vi "WPI_CameraSet Exposure Priority.vi"(8 "error in (no error)":errorcluster, 10 "Exposure Priority":T2, 11 "CameraDevRef":T1={"Camera Address"="192.168.0.90", "CameraStatus"={"status"=FALSE, "code"=0, "source"=""}}) -> (0 "error out":errorcluster, 3 "CameraDevRef Out":T1)   [LabVIEW 2017]
doc: "Specifies whether the camera you specify prioritizes the frame rate or image quality when setting the exposure.\n\nThis software is licensed. Open the labview\\readme\\WPI Robotics Library Open Source License.txt file for more information."
uses:
  <vilib>/Rock Robotics/WPI/Camera/WPI_CameraExposure Priority Values.ctl
  <vilib>/Rock Robotics/WPI/Camera/WPI_CameraDevRef.ctl
  <vilib>/Rock Robotics/WPI/Camera/WPI_CameraSettings Operations.ctl
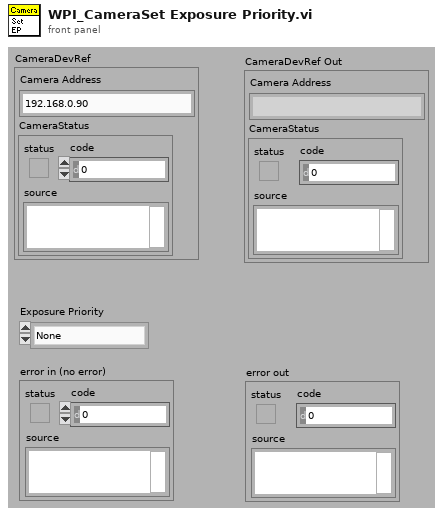
[diagram p1: front panel]
types:
  T1 = typedef "WPI_CameraDevRef.ctl" = cluster{"Camera Address":string, "CameraStatus":errorcluster}
  T2 = typedef "WPI_CameraExposure Priority Values.ctl" = enum16{"None", "Prioritize frame rate", "Prioritize image quality"}
  T3 = typedef "WPI_CameraSettings Operations.ctl" = enum16{"Udate FPS", "Update Compression", "Update Size", "Update White Balance", "Update Brightness", "Update Sharpness", "Update Exposure", "Update Exposure Value", "Update Color Level", "Update Exp Priority", "Update Color Enable", "Update JPG", "Update MJPG", "Read and Clear", "Read", "Init"}
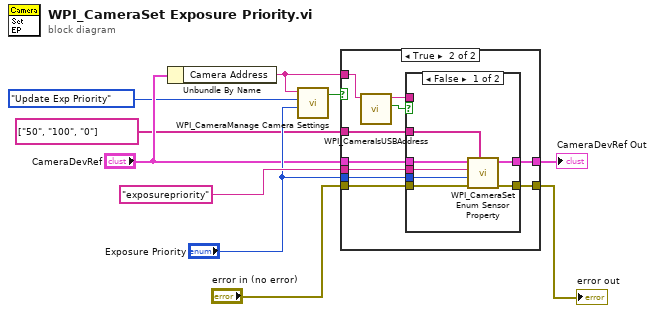
[diagram p0: block diagram]
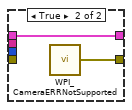
[diagram p3: hidden frame]
diagram:
  n1 = Unbundle By Name("CameraDevRef") -> ("Camera Address"=w2:string)
  n2 = call <vilib>:"WPI_CameraManage Camera Settings.vi"("Value"="Exposure Priority", "Operation"=WPI_CameraSettings_Operations."Update Exp Priority", "Camera IP"=w2) -> ("Changed"=w6:bool)  [unwired: 7 in, 1 out]
  n3 = case shown="True" w6 {
    tunnel: "CameraDevRef" -> [w11 w22]
    tunnel: "exposurepriority" ("Property Name") -> [_ w21]
    tunnel: string[] ["50", "100", "0"] -> [_ w20]
    tunnel: "Exposure Priority" -> [_ w19]
    tunnel: [w11 w18] -> w9
    tunnel: [w12 w17] -> w8
    tunnel: "error in (no error)" -> [w12 w16]
    tunnel: w2 -> [_ w15]
    frame False {
    }
    frame True {
      n4 = call <vilib>:"WPI_CameraIsUSBAddress.vi"("Camera Address In"=w15) -> ("USB?"=w14:bool, "Camera Address Out"=w13:string)  [unwired: 8 in, 1 out]
      n5 = case shown="False" w14 {
        tunnel: w22 -> [w29 w31]
        tunnel: w21 -> [w28 _]
        tunnel: w20 -> [w27 _]
        tunnel: w19 -> [w26 _]
        tunnel: [w25 w31] -> w18
        tunnel: [w24 w30] -> w17
        tunnel: w16 -> [w23 _]
        tunnel: w13 -> [_ _]
        frame False {
          n6 = call <vilib>:"WPI_CameraSet Enum Sensor Property.vi"("Strings"=w27, "error in (no error)"=w23, "Value"=w26, "Property Name"=w28, "CameraDevRef"=w29) -> ("error out"=w24:errorcluster, "CameraDevRef Out"=w25:T1)  [unwired: 5 out]
        }
        frame True {
          n7 = call <vilib>:"WPI_CameraERRNotSupported.vi"() -> ("error out"=w30:errorcluster)
        }
      }
    }
  }
  "CameraDevRef Out" <- w9
  "error out" <- w8
